vi "FGGA TCP Packet_v3.1.vi"(0 "ID":string, 5 "Version":string, 7 "TCP Packet In":string, 9 "utc_time":u32, 12 "Data Array":string[](array[string])) -> (8 "TCP Binary Packet":string)   [LabVIEW 2014]
panel:
  out "array":string[](array[string])
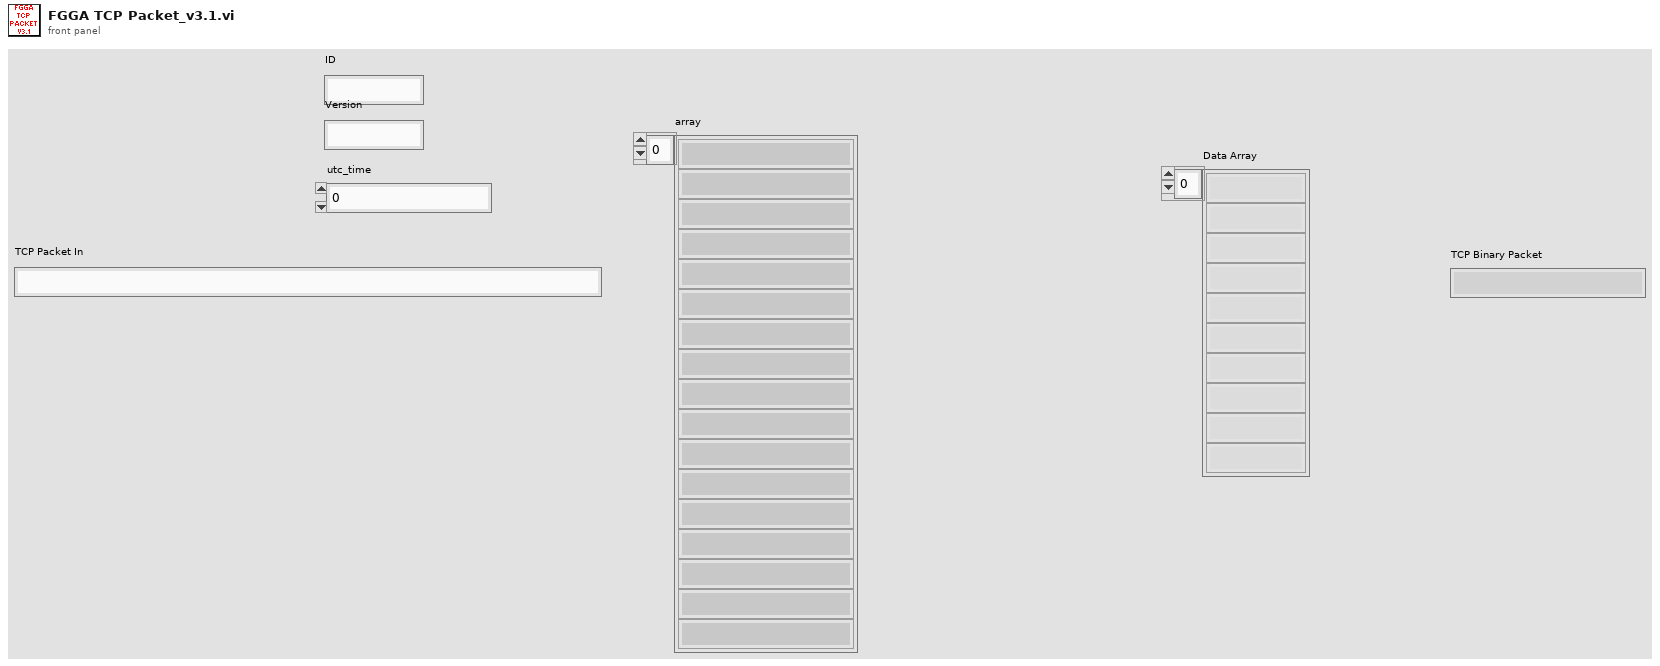
[diagram p1: front panel]
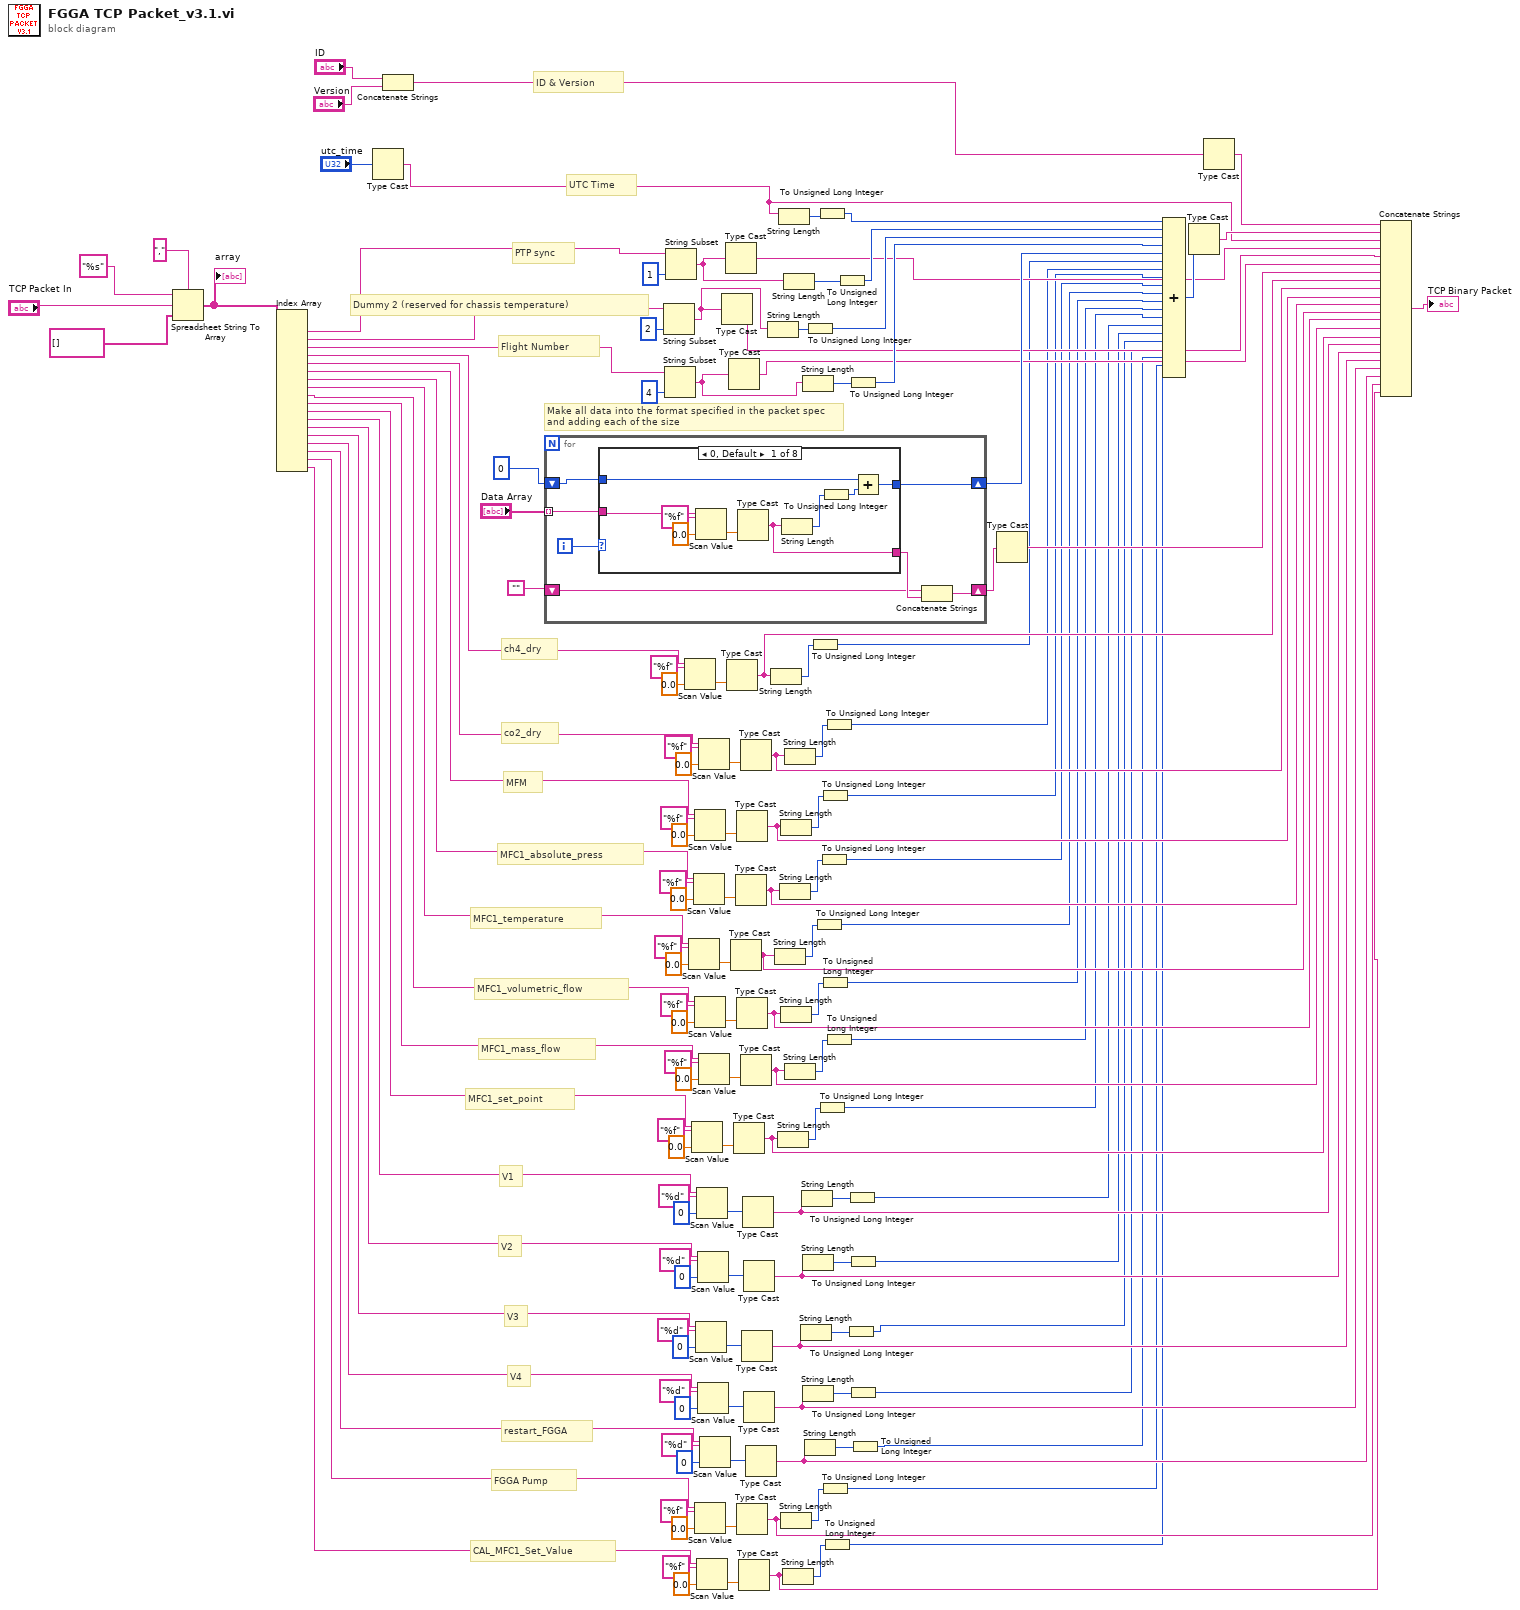
[diagram p0: block diagram]
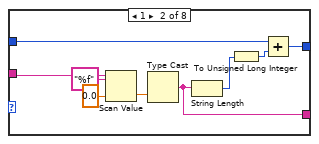
[diagram p2: hidden frame]
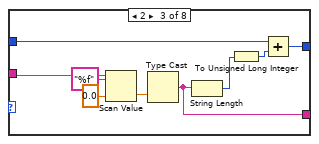
[diagram p3: hidden frame]
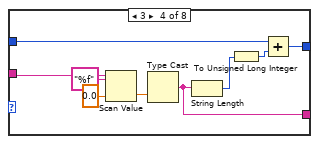
[diagram p4: hidden frame]
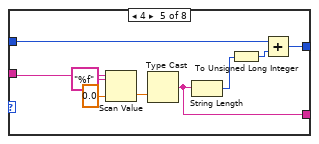
[diagram p5: hidden frame]
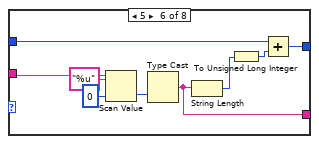
[diagram p6: hidden frame]
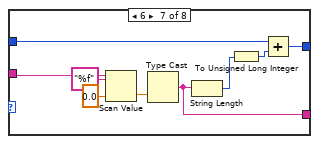
[diagram p7: hidden frame]
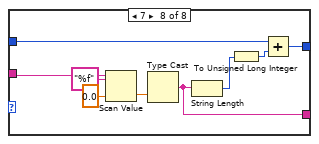
[diagram p8: hidden frame]
diagram:
  # "PTP sync"
  # "CAL_MFC1_Set_Value"
  # "FGGA Pump"
  # "restart_FGGA"
  # "V4"
  # "V3"
  # "V2"
  # "V1"
  # "MFC1_set_point"
  # "MFC1_mass_flow"
  # "MFC1_volumetric_flow"
  # "MFC1_temperature"
  # "MFC1_absolute_press"
  # "MFM"
  # "co2_dry"
  # "ch4_dry"
  # "Flight Number"
  # "Dummy 2 (reserved for chassis temperature)"
  # "UTC Time"
  # "ID & Version"
  # "Make all data into the format specified in the packet spec\nand adding each of the size"
  n1 = Spreadsheet String To Array(delimiter (Tab)=",", format string="%s", spreadsheet string="TCP Packet In", array type (2D Dbl)=string[] []) -> (array=w102:string[])
  "array" <- w102
  n2 = Index Array(array=w102) -> (element #1=w101:string, element #2=w100:string, element #3=w99:string, element #4=w98:string, element #5=w97:string, element #6=w72:string, element #7=w69:string, element #8=w66:string, element #9=w63:string, element #10=w60:string, element #11=w57:string, element #12=w50:string, element #13=w43:string, element #14=w20:string, element #15=w17:string, element #16=w14:string, element #17=w11:string, element #18=w8:string)  [unwired: 18 in]
  n3 = Type Cast(x="utc_time") -> (*(type *) &x=w1:string)  [unwired: 1 in]
  n4 = Concatenate Strings("ID", "Version") -> (w3:string)
  n5 = for {
    tunnel: "Data Array" -> [w151] mode=indexing
    shift-right: [w149] -> w133
    shift-left: u32 0 -> [w150]
    shift-right: [w148] -> w122
    shift-left: "" -> [w146]
    i -> [w152]
    n6 = case shown="0, Default" w152 {
      tunnel: w151 -> [w159 w168 w177 w186 w195 w204 w213 w222]
      tunnel: w150 -> [w157 w166 w175 w184 w193 w202 w211 w220]
      tunnel: [w154 w163 w172 w181 w190 w199 w208 w217] -> w149
      tunnel: [w153 w162 w171 w180 w189 w198 w207 w216] -> w147
      frame 0, Default {
        n7 = Scan Value(string=w159, format string="%f", default (0 dbl)=sgl 0.0 ("default (0 I32)")) -> (value=w161:sgl)  [unwired: 1 out]
        n8 = Type Cast(x=w161) -> (*(type *) &x=w153:string)  [unwired: 1 in]
        n9 = String Length(string=w153) -> (length=w156:i32)
        n10 = To Unsigned Long Integer(number=w156) -> (unsigned 32bit integer=w155:u32)
        n11 = Add(x=w157, y=w155) -> (x+y=w154:u32)
      }
      frame 1 {
        n12 = Scan Value(string=w168, format string="%f", default (0 dbl)=sgl 0.0 ("default (0 I32)")) -> (value=w170:sgl)  [unwired: 1 out]
        n13 = Type Cast(x=w170) -> (*(type *) &x=w162:string)  [unwired: 1 in]
        n14 = String Length(string=w162) -> (length=w165:i32)
        n15 = To Unsigned Long Integer(number=w165) -> (unsigned 32bit integer=w164:u32)
        n16 = Add(x=w166, y=w164) -> (x+y=w163:u32)
      }
      frame 2 {
        n17 = Scan Value(string=w177, format string="%f", default (0 dbl)=sgl 0.0 ("default (0 I32)")) -> (value=w179:sgl)  [unwired: 1 out]
        n18 = Type Cast(x=w179) -> (*(type *) &x=w171:string)  [unwired: 1 in]
        n19 = String Length(string=w171) -> (length=w174:i32)
        n20 = To Unsigned Long Integer(number=w174) -> (unsigned 32bit integer=w173:u32)
        n21 = Add(x=w175, y=w173) -> (x+y=w172:u32)
      }
      frame 3 {
        n22 = Scan Value(string=w186, format string="%f", default (0 dbl)=sgl 0.0 ("default (0 I32)")) -> (value=w188:sgl)  [unwired: 1 out]
        n23 = Type Cast(x=w188) -> (*(type *) &x=w180:string)  [unwired: 1 in]
        n24 = String Length(string=w180) -> (length=w183:i32)
        n25 = To Unsigned Long Integer(number=w183) -> (unsigned 32bit integer=w182:u32)
        n26 = Add(x=w184, y=w182) -> (x+y=w181:u32)
      }
      frame 4 {
        n27 = Scan Value(string=w195, format string="%f", default (0 dbl)=sgl 0.0 ("default (0 I32)")) -> (value=w197:sgl)  [unwired: 1 out]
        n28 = Type Cast(x=w197) -> (*(type *) &x=w189:string)  [unwired: 1 in]
        n29 = String Length(string=w189) -> (length=w192:i32)
        n30 = To Unsigned Long Integer(number=w192) -> (unsigned 32bit integer=w191:u32)
        n31 = Add(x=w193, y=w191) -> (x+y=w190:u32)
      }
      frame 5 {
        n32 = Scan Value(string=w204, format string="%u", default (0 dbl)=u16 0 ("default (0 I32)")) -> (value=w206:u16)  [unwired: 1 out]
        n33 = Type Cast(x=w206) -> (*(type *) &x=w198:string)  [unwired: 1 in]
        n34 = String Length(string=w198) -> (length=w201:i32)
        n35 = To Unsigned Long Integer(number=w201) -> (unsigned 32bit integer=w200:u32)
        n36 = Add(x=w202, y=w200) -> (x+y=w199:u32)
      }
      frame 6 {
        n37 = Scan Value(string=w213, format string="%f", default (0 dbl)=sgl 0.0 ("default (0 I32)")) -> (value=w215:sgl)  [unwired: 1 out]
        n38 = Type Cast(x=w215) -> (*(type *) &x=w207:string)  [unwired: 1 in]
        n39 = String Length(string=w207) -> (length=w210:i32)
        n40 = To Unsigned Long Integer(number=w210) -> (unsigned 32bit integer=w209:u32)
        n41 = Add(x=w211, y=w209) -> (x+y=w208:u32)
      }
      frame 7 {
        n42 = Scan Value(string=w222, format string="%f", default (0 dbl)=sgl 0.0 ("default (0 I32)")) -> (value=w224:sgl)  [unwired: 1 out]
        n43 = Type Cast(x=w224) -> (*(type *) &x=w216:string)  [unwired: 1 in]
        n44 = String Length(string=w216) -> (length=w219:i32)
        n45 = To Unsigned Long Integer(number=w219) -> (unsigned 32bit integer=w218:u32)
        n46 = Add(x=w220, y=w218) -> (x+y=w217:u32)
      }
    }
    n47 = Concatenate Strings(w146, w147) -> (w148:string)
  }
  n48 = String Subset(string=w100, length (rest)=2 ("length (rest)")) -> (substring=w120:string)  [unwired: 1 in]
  n49 = String Subset(string=w99, length (rest)=4 ("length (rest)")) -> (substring=w126:string)  [unwired: 1 in]
  n50 = String Subset(string=w101, length (rest)=1 ("length (rest)")) -> (substring=w129:string)  [unwired: 1 in]
  n51 = Scan Value(string=w98, format string="%f", default (0 dbl)=sgl 0.0 ("default (0 I32)")) -> (value=w118:sgl)  [unwired: 1 out]
  n52 = Scan Value(string=w66, format string="%f", default (0 dbl)=sgl 0.0 ("default (0 I32)")) -> (value=w88:sgl)  [unwired: 1 out]
  n53 = Scan Value(string=w57, format string="%f", default (0 dbl)=sgl 0.0 ("default (0 I32)")) -> (value=w76:sgl)  [unwired: 1 out]
  n54 = Scan Value(string=w69, format string="%f", default (0 dbl)=sgl 0.0 ("default (0 I32)")) -> (value=w92:sgl)  [unwired: 1 out]
  n55 = Scan Value(string=w72, format string="%f", default (0 dbl)=sgl 0.0 ("default (0 I32)")) -> (value=w96:sgl)  [unwired: 1 out]
  n56 = Scan Value(string=w63, format string="%f", default (0 dbl)=sgl 0.0 ("default (0 I32)")) -> (value=w84:sgl)  [unwired: 1 out]
  n57 = Scan Value(string=w11, format string="%f", default (0 dbl)=sgl 0.0 ("default (0 I32)")) -> (value=w28:sgl)  [unwired: 1 out]
  n58 = Scan Value(string=w20, format string="%d", default (0 dbl)=u16 0 ("default (0 I32)")) -> (value=w37:u16)  [unwired: 1 out]
  n59 = Scan Value(string=w50, format string="%d", default (0 dbl)=u16 0 ("default (0 I32)")) -> (value=w51:u16)  [unwired: 1 out]
  n60 = Scan Value(string=w8, format string="%f", default (0 dbl)=sgl 0.0 ("default (0 I32)")) -> (value=w24:sgl)  [unwired: 1 out]
  n61 = Scan Value(string=w43, format string="%d", default (0 dbl)=u16 0 ("default (0 I32)")) -> (value=w44:u16)  [unwired: 1 out]
  n62 = Scan Value(string=w17, format string="%d", default (0 dbl)=u16 0 ("default (0 I32)")) -> (value=w33:u16)  [unwired: 1 out]
  n63 = Scan Value(string=w97, format string="%f", default (0 dbl)=sgl 0.0 ("default (0 I32)")) -> (value=w112:sgl)  [unwired: 1 out]
  n64 = Scan Value(string=w60, format string="%f", default (0 dbl)=sgl 0.0 ("default (0 I32)")) -> (value=w80:sgl)  [unwired: 1 out]
  n65 = Scan Value(string=w14, format string="%d", default (0 dbl)=u16 0 ("default (0 I32)")) -> (value=w29:u16)  [unwired: 1 out]
  n66 = Type Cast(x=w120) -> (*(type *) &x=w119:string)  [unwired: 1 in]
  n67 = Type Cast(x=w129) -> (*(type *) &x=w128:string)  [unwired: 1 in]
  n68 = Type Cast(x=w118) -> (*(type *) &x=w114:string)  [unwired: 1 in]
  n69 = Type Cast(x=w126) -> (*(type *) &x=w127:string)  [unwired: 1 in]
  n70 = Type Cast(x=w88) -> (*(type *) &x=w64:string)  [unwired: 1 in]
  n71 = Type Cast(x=w76) -> (*(type *) &x=w55:string)  [unwired: 1 in]
  n72 = Type Cast(x=w92) -> (*(type *) &x=w67:string)  [unwired: 1 in]
  n73 = Type Cast(x=w96) -> (*(type *) &x=w70:string)  [unwired: 1 in]
  n74 = Type Cast(x=w84) -> (*(type *) &x=w61:string)  [unwired: 1 in]
  n75 = Type Cast(x=w28) -> (*(type *) &x=w9:string)  [unwired: 1 in]
  n76 = Type Cast(x=w24) -> (*(type *) &x=w6:string)  [unwired: 1 in]
  n77 = Type Cast(x=w112) -> (*(type *) &x=w107:string)  [unwired: 1 in]
  n78 = Type Cast(x=w80) -> (*(type *) &x=w58:string)  [unwired: 1 in]
  n79 = Type Cast(x=w37) -> (*(type *) &x=w18:string)  [unwired: 1 in]
  n80 = Type Cast(x=w51) -> (*(type *) &x=w48:string)  [unwired: 1 in]
  n81 = Type Cast(x=w44) -> (*(type *) &x=w41:string)  [unwired: 1 in]
  n82 = Type Cast(x=w33) -> (*(type *) &x=w15:string)  [unwired: 1 in]
  n83 = Type Cast(x=w29) -> (*(type *) &x=w12:string)  [unwired: 1 in]
  n84 = String Length(string=w120) -> (length=w140:i32)
  n85 = String Length(string=w114) -> (length=w115:i32)
  n86 = String Length(string=w64) -> (length=w85:i32)
  n87 = String Length(string=w55) -> (length=w73:i32)
  n88 = String Length(string=w1) -> (length=w145:i32)
  n89 = String Length(string=w67) -> (length=w89:i32)
  n90 = String Length(string=w70) -> (length=w93:i32)
  n91 = String Length(string=w61) -> (length=w81:i32)
  n92 = String Length(string=w9) -> (length=w25:i32)
  n93 = String Length(string=w6) -> (length=w21:i32)
  n94 = String Length(string=w129) -> (length=w142:i32)
  n95 = String Length(string=w107) -> (length=w109:i32)
  n96 = String Length(string=w58) -> (length=w77:i32)
  n97 = String Length(string=w18) -> (length=w40:i32)
  n98 = String Length(string=w48) -> (length=w54:i32)
  n99 = String Length(string=w126) -> (length=w137:i32)
  n100 = String Length(string=w41) -> (length=w47:i32)
  n101 = String Length(string=w15) -> (length=w36:i32)
  n102 = To Unsigned Long Integer(number=w140) -> (unsigned 32bit integer=w139:u32)
  n103 = String Length(string=w12) -> (length=w32:i32)
  n104 = To Unsigned Long Integer(number=w115) -> (unsigned 32bit integer=w113:u32)
  n105 = To Unsigned Long Integer(number=w85) -> (unsigned 32bit integer=w65:u32)
  n106 = To Unsigned Long Integer(number=w145) -> (unsigned 32bit integer=w144:u32)
  n107 = To Unsigned Long Integer(number=w73) -> (unsigned 32bit integer=w56:u32)
  n108 = To Unsigned Long Integer(number=w89) -> (unsigned 32bit integer=w68:u32)
  n109 = To Unsigned Long Integer(number=w93) -> (unsigned 32bit integer=w71:u32)
  n110 = To Unsigned Long Integer(number=w81) -> (unsigned 32bit integer=w62:u32)
  n111 = To Unsigned Long Integer(number=w25) -> (unsigned 32bit integer=w10:u32)
  n112 = To Unsigned Long Integer(number=w21) -> (unsigned 32bit integer=w7:u32)
  n113 = To Unsigned Long Integer(number=w109) -> (unsigned 32bit integer=w108:u32)
  n114 = To Unsigned Long Integer(number=w77) -> (unsigned 32bit integer=w59:u32)
  n115 = To Unsigned Long Integer(number=w142) -> (unsigned 32bit integer=w141:u32)
  n116 = To Unsigned Long Integer(number=w40) -> (unsigned 32bit integer=w19:u32)
  n117 = To Unsigned Long Integer(number=w54) -> (unsigned 32bit integer=w49:u32)
  n118 = To Unsigned Long Integer(number=w137) -> (unsigned 32bit integer=w136:u32)
  n119 = To Unsigned Long Integer(number=w47) -> (unsigned 32bit integer=w42:u32)
  n120 = To Unsigned Long Integer(number=w36) -> (unsigned 32bit integer=w16:u32)
  n121 = To Unsigned Long Integer(number=w32) -> (unsigned 32bit integer=w13:u32)
  n122 = Type Cast(x=w122) -> (*(type *) &x=w125:string)  [unwired: 1 in]
  n123 = Compound Arithmetic op=ADD(w144, w141, w139, w136, w133, w113, w108, w71, w68, w65, w62, w59, w56, w49, w42, w19, w16, w13, w10, w7) -> (w131:u32)
  n124 = Type Cast(x=w131) -> (*(type *) &x=w130:string)  [unwired: 1 in]
  n125 = Type Cast(x=w3) -> (*(type *) &x=w132:string)  [unwired: 1 in]
  n126 = Concatenate Strings(w132, w130, w1, w128, w119, w127, w125, w114, w107, w70, w67, w64, w61, w58, w55, w48, w41, w18, w15, w12, w9, w6) -> (→"TCP Binary Packet":string)
